vi "可重入.vi"() -> ()   [LabVIEW 2013]
panel:
  out "属于副本VI":bool
  out "VI副本名":string
  out "VI名称":string
  out "VI路径":path
  in  "停止":bool
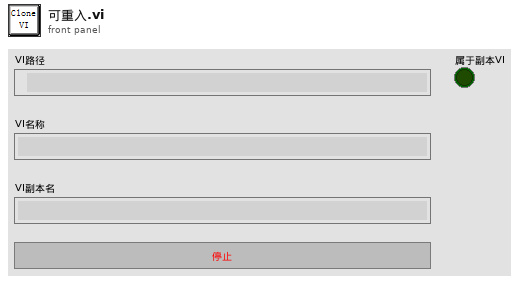
[diagram p1: front panel]
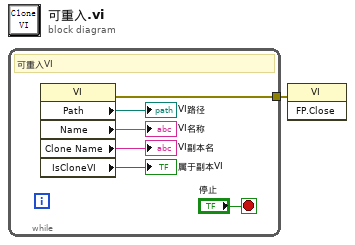
[diagram p0: block diagram]
diagram:
  n1 = while {
    tunnel: [w3] -> w1
    stop <- "停止" stop-if-true
    # "可重入VI"
    n2 = property class="VI"() -> (error out=w3:errorcluster, "Path"=→"VI路径":path, "Name"=→"VI名称":string, "Clone Name"=→"VI副本名":string, "IsCloneVI"=→"属于副本VI":bool)  [unwired: 2 in, 1 out]
  }
  n3 = invoke class="VI" method="FP.Close"(error in=w1) -> ()  [unwired: 2 in, 3 out]
